vi "Extract_Data_TCP.vi"(8 "error in (no error)":errorcluster, 10 "Data Recieved":u8[](array[numeric]) format="%.0x", 11 "Siemens Ctr in":T1) -> (0 "error out":errorcluster, 1 "PDU Exchanged":bool, 2 "Message Error":u16, 3 "Siemens Ctr":T1, 4 "Data Valid":bool, 5 "Data":u8[](array[numeric]), 6 "Error Code":u8)   [LabVIEW 2014, in "Simatic S7.lvlib"]
uses:
  Simatic S7.lvlib
panel:
  out "Length in Bytes":u16
  out "Data Transport Size":u8
  out "Returning Write Data":bool
  out "Number of Items Read":u8
  out "Returning Read Data":bool
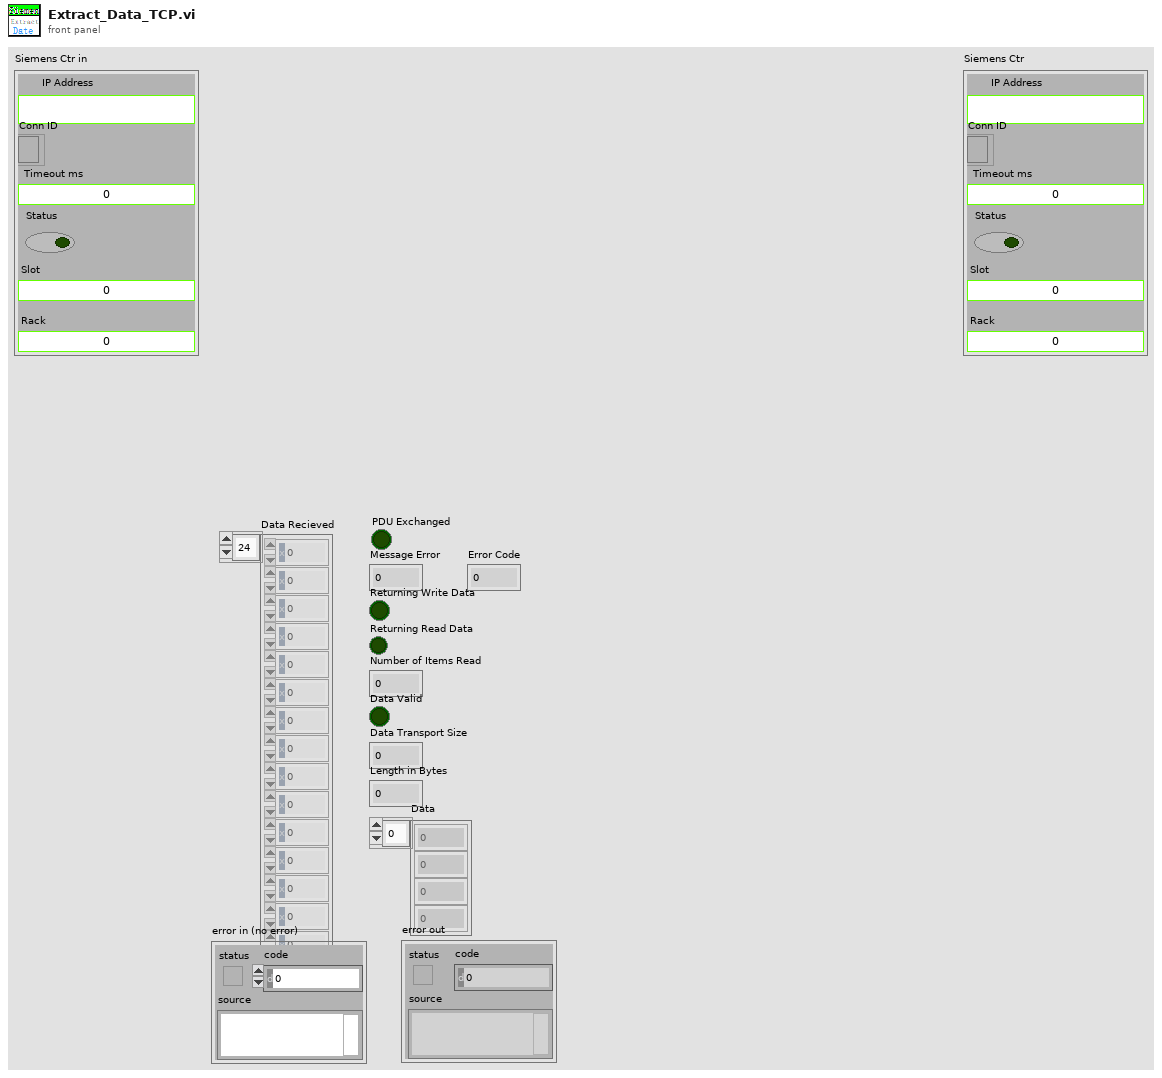
[diagram p1: front panel]
types:
  T1 = typedef "Simatic S7.lvlib/Siemens Ref.ctl" = cluster{"IP Address ":string, "Conn ID":refnum<k5>, "Timeout ms":i32, "Status":bool, "Slot":u16, "Rack":u16}
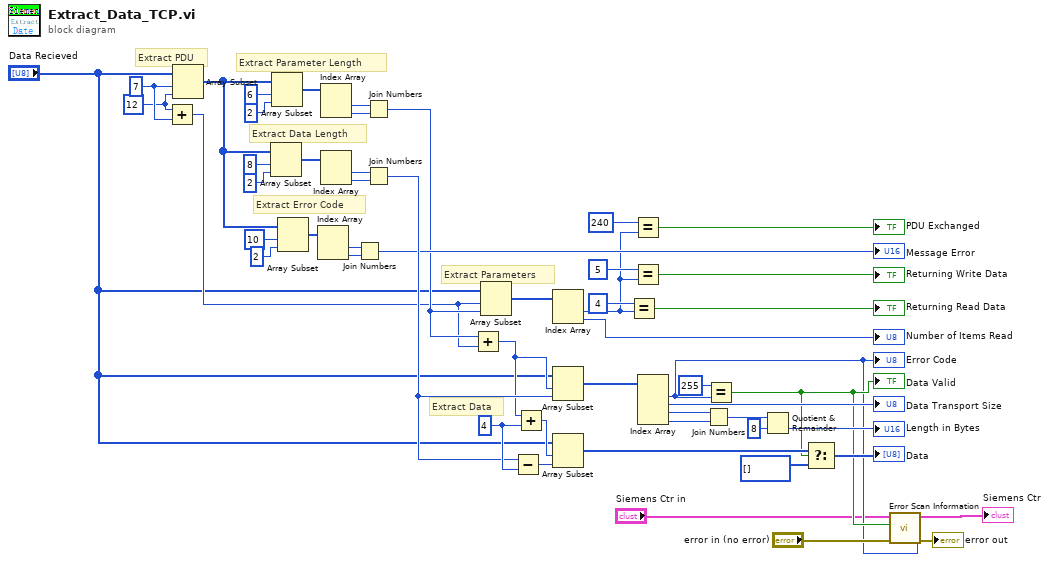
[diagram p0: block diagram]
diagram:
  w53 = 4 ("y")
  w12 = 12 ("length")
  w13 = 7 ("index")
  # "Extract Error Code"
  # "Extract Parameters"
  # "Extract Data"
  # "Extract Data Length"
  # "Extract Parameter Length"
  # "Extract PDU"
  n1 = Add(x=w12, y=w13) -> (x+y=w11:i32)
  n2 = Array Subset(array="Data Recieved", index=w13, length=w12) -> (w26:u8[])
  n3 = Array Subset(array=w26, index=8, length=2) -> (w32:u8[])
  n4 = Array Subset(array=w26, index=6, length=2) -> (w27:u8[])
  n5 = Array Subset(array=w26, index=10, length=2) -> (w46:u8[])
  n6 = Index Array(array=w46) -> (element #1=w43:u8, element #2=w47:u8)  [unwired: 2 in]
  n7 = Index Array(array=w27) -> (element #1=w28:u8, element #2=w29:u8)  [unwired: 2 in]
  n8 = Index Array(array=w32) -> (element #1=w31:u8, element #2=w30:u8)  [unwired: 2 in]
  n9 = Join Numbers(hi=w43, lo=w47) -> ((hi.lo)=→"Message Error":u16)
  n10 = Join Numbers(hi=w28, lo=w29) -> ((hi.lo)=w33:u16)
  n11 = Join Numbers(hi=w31, lo=w30) -> ((hi.lo)=w52:u16)
  n12 = Add(x=w33, y=w11) -> (x+y=w48:i32)
  n13 = Array Subset(array="Data Recieved", index=w11, length=w33) -> (w34:u8[])
  n14 = Subtract(x=w52, y=w53) -> (x-y=w51:i32)
  n15 = Add(x=w48, y=w53) -> (x+y=w50:i32)
  n16 = Index Array(array=w34) -> (element #1=w15:u8, element #2=→"Number of Items Read":u8)  [unwired: 2 in]
  n17 = Array Subset(array="Data Recieved", index=w48, length=w52) -> (w49:u8[])
  n18 = Array Subset(array="Data Recieved", index=w50, length=w51) -> (w9:u8[])
  n19 = Equal?(x=u8 4, y=w15) -> (x = y?=→"Returning Read Data":bool)
  n20 = Equal?(x=u8 240, y=w15) -> (x = y?=→"PDU Exchanged":bool)
  n21 = Equal?(x=u8 5, y=w15) -> (x = y?=→"Returning Write Data":bool)
  n22 = Index Array(array=w49) -> (element #1=w4:u8, element #2=→"Data Transport Size":u8, element #3=w40:u8, element #4=w41:u8)  [unwired: 4 in]
  "Error Code" <- w4
  n23 = Join Numbers(hi=w40, lo=w41) -> ((hi.lo)=w19:u16)
  n24 = Equal?(x=u8 255, y=w4) -> (x = y?=w5:bool)
  "Data Valid" <- w5
  n25 = Quotient & Remainder(x=w19, y=u16 8) -> (floor(x/y)=→"Length in Bytes":u16)  [unwired: 1 out]
  n26 = Select(t=w9, s=w5, f=u8[] []) -> (s? t:f=→"Data":u8[])
  n27 = call "Error Scan Information.vi"("Error Code"=w4, "error in (no error)"="error in (no error)", "Data Valid"=w5, "Siemens Ctr"="Siemens Ctr in") -> ("error out"=→"error out":errorcluster, "Siemens Ctr out"=→"Siemens Ctr":T1)  [unwired: 6 in]
